vi "Read 1x160 Voltage Map.vi"(8 "error in (no error)":errorcluster, 11 "BMC in":refnum<class "BMC.lvclass">) -> (0 "error out":errorcluster, 2 "1x160  Voltage Map":dbl[](array[numeric]), 3 "BMC out":refnum<class "BMC.lvclass">)   [LabVIEW 2012, in "BMC.lvclass"]
uses:
  BMC.lvclass
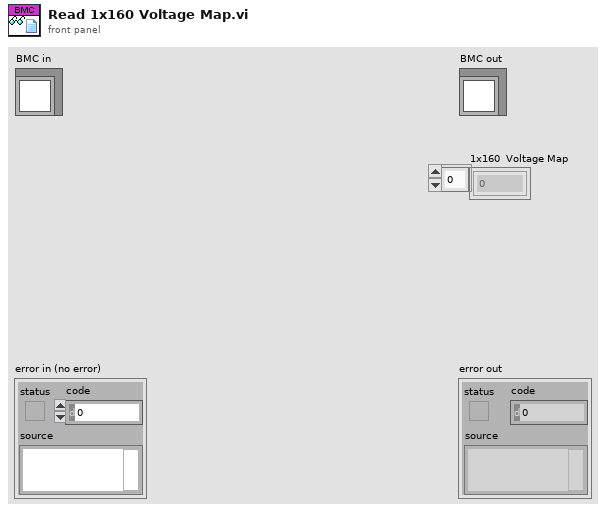
[diagram p1: front panel]
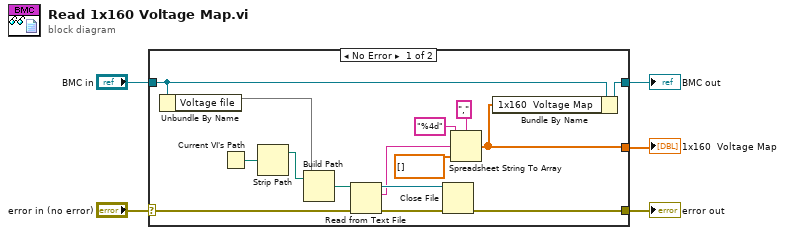
[diagram p0: block diagram]
diagram:
  n1 = case shown="No Error" "error in (no error)" {
    selector: "error in (no error)" -> [w15 w22]
    tunnel: [w14 w22] -> w4
    tunnel: [w13 w21] -> w2
    tunnel: "BMC in" -> [w7 w21]
    tunnel: [w9 _] -> w1
    frame No Error {
      n2 = Unbundle By Name(w7) -> ("Voltage file"=w6)
      n3 = Current VI's Path() -> (path=w11:path)
      n4 = Strip Path(path=w11) -> (stripped path=w12:path)  [unwired: 1 out]
      n5 = Build Path(base path=w12, name or relative path=w6) -> (appended path=w10:path)
      n6 = Read from Text File(file (use dialog)=w10, error in=w15) -> (refnum out=w20:refnum<file>, text=w18:string, error out=w19:errorcluster)  [unwired: 3 out]
      n7 = Close File(refnum=w20, error in=w19) -> (error out=w14:errorcluster)  [unwired: 1 out]
      n8 = Spreadsheet String To Array(delimiter (Tab)=",", format string="%4d", spreadsheet string=w18, array type (2D Dbl)=dbl[] [] ("settings_cluster.1x160  Voltage Map")) -> (array=w9:dbl[])
      n9 = Bundle By Name(cluster=w7, "1x160  Voltage Map"=w9) -> (w13:refnum<class "BMC.lvclass">)
    }
    frame Error {
    }
  }
  "error out" <- w4
  "BMC out" <- w2
  "1x160  Voltage Map" <- w1
